vi "ContinuosSplitMicroSettings.vi"(0 "Loop Microscope Settings":string[][](array[string])) -> (4 "Objective":i32[](array[numeric]), 6 "Filter":string[](array[string]), 8 "Exposure Time":i32[](array[numeric]), 10 "Prism":string[](array[string]), 15 "Intensity":dbl[](array[numeric]))   [LabVIEW 2018]
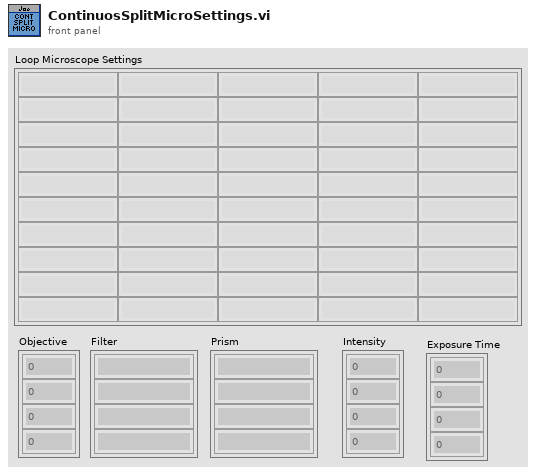
[diagram p1: front panel]
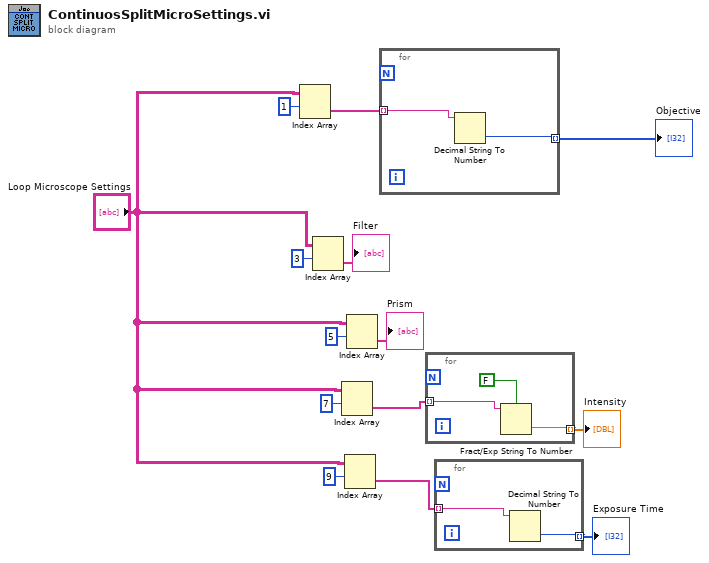
[diagram p0: block diagram]
diagram:
  n1 = Index Array(array="Loop Microscope Settings", index (row)=1) -> (element=w13:string[])  [unwired: 1 in]
  n2 = Index Array(array="Loop Microscope Settings", index (row)=3) -> (element=→"Filter":string[])  [unwired: 1 in]
  n3 = Index Array(array="Loop Microscope Settings", index (row)=7) -> (element=w3:string[])  [unwired: 1 in]
  n4 = Index Array(array="Loop Microscope Settings", index (row)=9) -> (element=w4:string[])  [unwired: 1 in]
  n5 = Index Array(array="Loop Microscope Settings", index (row)=5) -> (element=→"Prism":string[])  [unwired: 1 in]
  n6 = for {
    tunnel: w13 -> [w16] mode=indexing
    tunnel: [w15] -> w12 mode=indexing
    n7 = Decimal String To Number(string=w16) -> (number=w15:i32)  [unwired: 2 in, 1 out]
  }
  "Objective" <- w12
  n8 = for {
    tunnel: w3 -> [w19] mode=indexing
    tunnel: [w18] -> w2 mode=indexing
    n9 = Fract/Exp String To Number(use system decimal point (T)=FALSE, string=w19) -> (number=w18:dbl)  [unwired: 2 in, 1 out]
  }
  "Intensity" <- w2
  n10 = for {
    tunnel: w4 -> [w21] mode=indexing
    tunnel: [w20] -> w1 mode=indexing
    n11 = Decimal String To Number(string=w21) -> (number=w20:i32)  [unwired: 2 in, 1 out]
  }
  "Exposure Time" <- w1
